vi "LVPortSetObjectMapNamepathDataToVartiant.vi"(0 "Type (or value to update)":variant, 1 "MatlabDataBundle":T1, 2 "NamePath":string[](array[string]), 3 "Namepath Index":i32, 6 "Allow Variant Values (f)":bool, 18 "Info":string[](array[string])) -> (14 "Value":variant)   [LabVIEW 2017]
uses:
  LVPortObjectMapNamepathData.ctl
  LVPortObjectMapDataTypeEnum.ctl
  LVPortObjectMapContainerTypeEnum.ctl
panel:
  out "Updating index":i32
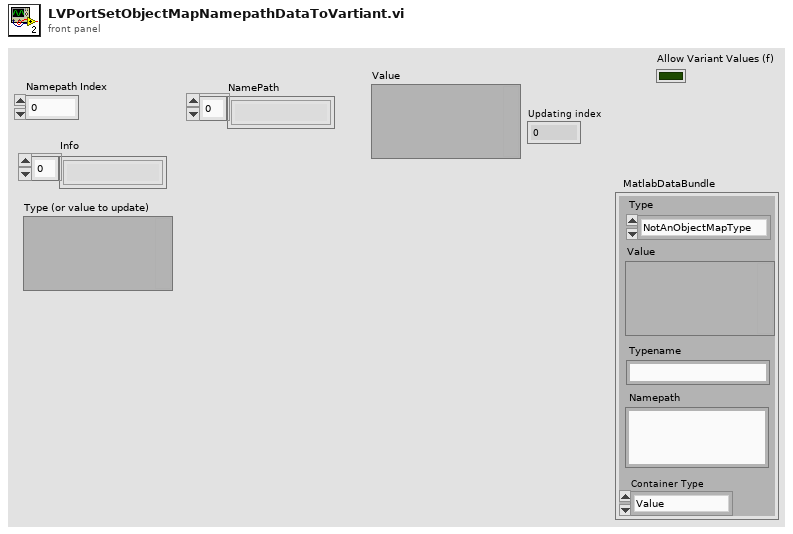
[diagram p1: front panel]
types:
  T1 = typedef "LVPortObjectMapNamepathData.ctl" = cluster{"Type":T2, "Value":variant, "Namepath":string, "Typename":string, "Container Type":T3}
  T2 = typedef "LVPortObjectMapDataTypeEnum.ctl" = enum16{"NotAnObjectMapType", "Real", "Complex", "String", "Boolean"}
  T3 = typedef "LVPortObjectMapContainerTypeEnum.ctl" = enum16{"Value", "Array", "Waveform"}
  T4 = typedef "NI_Data Type.lvlib/Data Type.ctl" = enum8{"Invalid Type", "Void", "I8", "I16", "I32", "I64", "U8", "U16", "U32", "U64", "Single Float", "Double Float", "Extended Float", "Single Complex", "Double Complex", "Extended Complex", "Enum U8", "Enum U16", "Enum U32", "Enum U64", "Single Float With Unit", "Double Float With Unit", "Extended Float With Unit", "Single Complex with Unit", "Double Complex with Unit", "Extended Complex with Unit", "Boolean", "String", "Path", "Picture", "Tag", "Array", "Cluster", "Variant", "LV Variant", "Waveform", "Timestamp", "Digital Waveform", "Digital Data", "ExpressData", "Refnum", "External Data", "VI", "Poly VI", "LabVIEW Class Instance", "Fixed Point"}
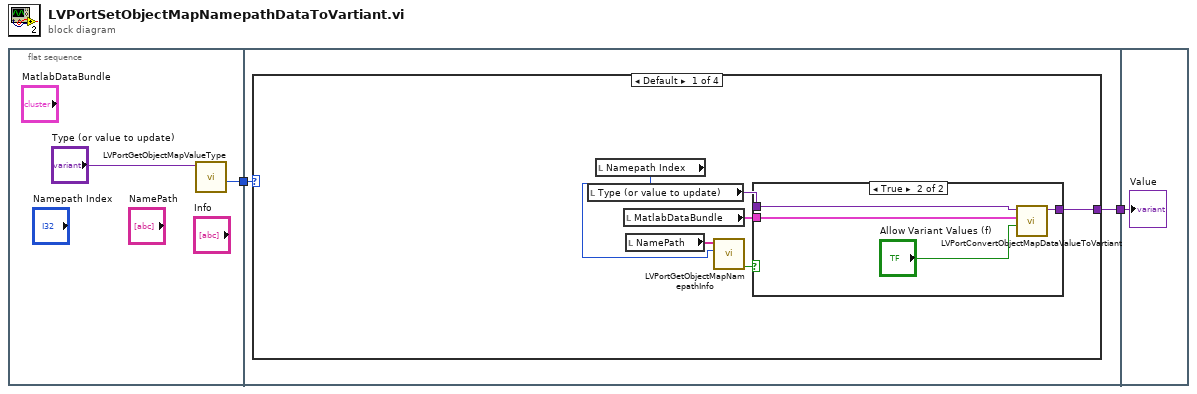
[diagram p0: block diagram]
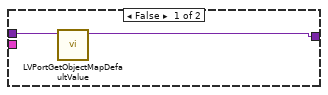
[diagram p2: hidden frame]
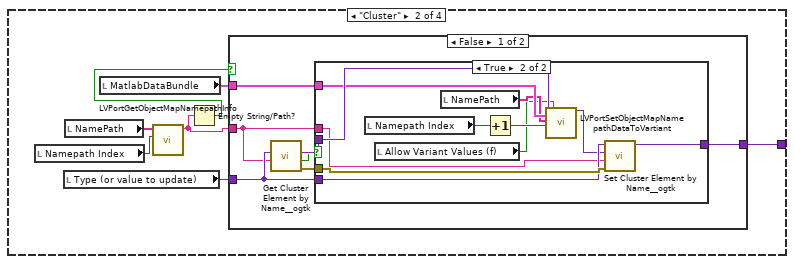
[diagram p3: hidden frame]
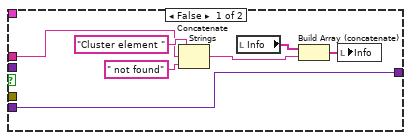
[diagram p4: hidden frame]
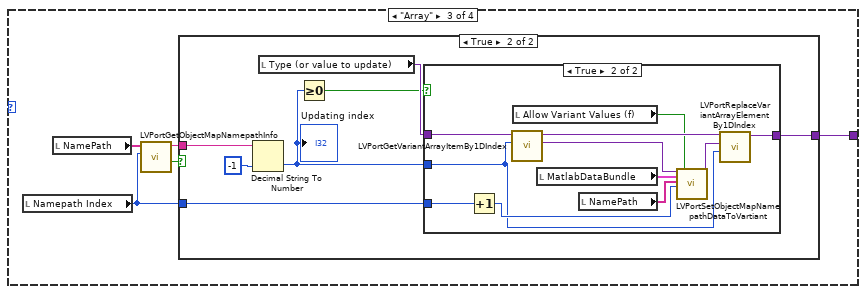
[diagram p6: hidden frame]
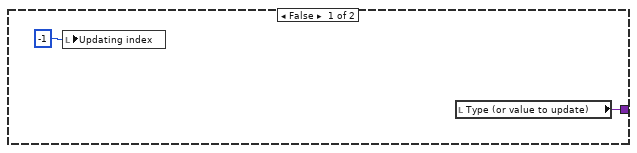
[diagram p7: hidden frame]
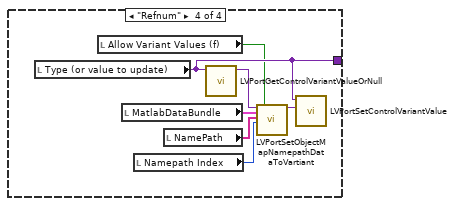
[diagram p9: hidden frame]
diagram:
  n1 = flat-sequence {
    tunnel: [w3] -> w2
    tunnel: w2 -> [w5]
    tunnel: [w6] -> w1
    tunnel: w1 -> [w85]
    frame #0 {
      n2 = call "LVPortGetObjectMapValueType.vi"("Value"="Type (or value to update)") -> ("Type"=w3:T4)  [unwired: 6 in, 4 out]
    }
    frame #1 {
      n3 = case shown="Default" w5 {
        tunnel: [w12 w23 w56 w82] -> w6
        frame Default {
          n4 = local read "Type (or value to update)"() -> (w11:variant)
          n5 = local read "Namepath Index"() -> (w9:i32)
          n6 = local read "MatlabDataBundle"() -> (w10:T1)
          n7 = local read "NamePath"() -> (w8:string[])
          n8 = call "LVPortGetObjectMapNamepathInfo.vi"("Namepath Index"=w9, "NamePath"=w8) -> ("At path end"=w7:bool)  [unwired: 7 in, 2 out]
          n9 = case shown="True" w7 {
            tunnel: [w14 w18] -> w12
            tunnel: w11 -> [w13 w17]
            tunnel: w10 -> [_ w16]
            frame False {
              n10 = call "LVPortGetObjectMapDefaultValue.vi"("From Value Type"=w13) -> ("Default Value"=w14:variant)  [unwired: 10 in]
            }
            frame True {
              n11 = call "LVPortConvertObjectMapDataValueToVartiant.vi"("Allow Variant Values (f)"="Allow Variant Values (f)", "MatlabDataBundle"=w16, "Data Value"=w17) -> ("Value"=w18:variant)  [unwired: 8 in]
            }
          }
        }
        frame "Cluster" {
          n12 = local read "Namepath Index"() -> (w19:i32)
          n13 = local read "Type (or value to update)"() -> (w24:variant)
          n14 = local read "NamePath"() -> (w21:string[])
          n15 = local read "MatlabDataBundle"() -> (w25:T1)
          n16 = call "LVPortGetObjectMapNamepathInfo.vi"("Namepath Index"=w19, "NamePath"=w21) -> ("Name"=w20:string)  [unwired: 7 in, 2 out]
          n17 = Empty String/Path?(string/path=w20) -> (empty?=w22:bool)
          n18 = case shown="False" w22 {
            tunnel: w25 -> [w31 _]
            tunnel: w24 -> [w29 w51]
            tunnel: [w28 w51] -> w23
            tunnel: w20 -> [w27 _]
            frame False {
              n19 = call <userlib>:"Get Cluster Element by Name__ogtk.vi"("Element Name"=w27, "Cluster"=w29) -> ("error out"=w30:errorcluster, "found?"=w26:bool, "VElement"=w32:variant)  [unwired: 7 in]
              n20 = case shown="True" w26 {
                tunnel: w32 -> [_ w50]
                tunnel: w31 -> [_ w49]
                tunnel: w30 -> [_ w48]
                tunnel: w29 -> [w39 w47]
                tunnel: [w39 w46] -> w28
                tunnel: w27 -> [w35 w44]
                frame False {
                  n21 = Concatenate Strings("Cluster element ", w35, " not found") -> (w37:string)
                  n22 = local read "Info"() -> (w38:string[])
                  n23 = Build Array (concatenate)(w38, w37) -> (w33:string[])
                  n24 = local write "Info"(w33) -> ()
                }
                frame True {
                  n25 = local read "Namepath Index"() -> (w42:i32)
                  n26 = local read "Allow Variant Values (f)"() -> (w40:bool)
                  n27 = local read "NamePath"() -> (w43:string[])
                  n28 = Increment(x=w42) -> (x+1=w41:i32)
                  n29 = call "LVPortSetObjectMapNamepathDataToVartiant.vi"("Type (or value to update)"=w50, "MatlabDataBundle"=w49, "NamePath"=w43, "Namepath Index"=w41, "Allow Variant Values (f)"=w40) -> ("Value"=w45:variant)  [unwired: 14 in]
                  n30 = call <userlib>:"Set Cluster Element by Name__ogtk.vi"("error in (no error)"=w48, "Element Name (\"\": New Element Data Name)"=w44, "New Element Value"=w45, "Cluster"=w47) -> ("VCluster out"=w46:variant)  [unwired: 5 in, 2 out]
                }
              }
            }
            frame True {
            }
          }
        }
        frame "Array" {
          n31 = local read "Namepath Index"() -> (w55:i32)
          n32 = local read "NamePath"() -> (w54:string[])
          n33 = call "LVPortGetObjectMapNamepathInfo.vi"("Namepath Index"=w55, "NamePath"=w54) -> ("Namepart found?"=w52:bool, "Name"=w53:string)  [unwired: 7 in, 1 out]
          n34 = case shown="True" w52 {
            tunnel: [w58 w64] -> w56
            tunnel: w55 -> [_ w60]
            tunnel: w53 -> [_ w59]
            frame False {
              n35 = local write "Updating index"(-1 ("Updating index")) -> ()
              n36 = local read "Type (or value to update)"() -> (w58:variant)
            }
            frame True {
              n37 = Decimal String To Number(string=w59, default (0L)=-1 ("default (0 I32)")) -> (number=w62:i32)  [unwired: 1 in, 1 out]
              "Updating index" <- w62
              n38 = local read "Type (or value to update)"() -> (w65:variant)
              n39 = Greater Or Equal To 0?(x=w62) -> (x >= 0?=w61:bool)
              n40 = case shown="True" w61 {
                tunnel: w65 -> [w66 w77]
                tunnel: w62 -> [_ w68]
                tunnel: [w66 w71] -> w64
                tunnel: w60 -> [_ w70]
                frame False {
                }
                frame True {
                  n41 = Increment(x=w70) -> (x+1=w69:i32)
                  n42 = call "LVPortGetVariantArrayItemBy1DIndex.vi"("Index"=w68, "Array in"=w77) -> ("Array Element"=w74:variant, "Array out"=w72:variant)  [unwired: 8 in]
                  n43 = local read "Allow Variant Values (f)"() -> (w67:bool)
                  n44 = local read "MatlabDataBundle"() -> (w75:T1)
                  n45 = local read "NamePath"() -> (w76:string[])
                  n46 = call "LVPortSetObjectMapNamepathDataToVartiant.vi"("Type (or value to update)"=w74, "MatlabDataBundle"=w75, "NamePath"=w76, "Namepath Index"=w69, "Allow Variant Values (f)"=w67) -> ("Value"=w73:variant)  [unwired: 14 in]
                  n47 = call "LVPortReplaceVariantArrayElementBy1DIndex.vi"("Index (1D)"=w68, "Value"=w73, "Array in"=w72) -> ("Array out"=w71:variant)  [unwired: 8 in]
                }
              }
            }
          }
        }
        frame "Refnum" {
          n48 = local read "Type (or value to update)"() -> (w82:variant)
          n49 = local read "Allow Variant Values (f)"() -> (w78:bool)
          n50 = local read "MatlabDataBundle"() -> (w81:T1)
          n51 = local read "Namepath Index"() -> (w79:i32)
          n52 = local read "NamePath"() -> (w80:string[])
          n53 = call "LVPortGetControlVariantValueOrNull.vi"("ControlVariant"=w82) -> ("Value"=w84:variant)  [unwired: 9 in, 1 out]
          n54 = call "LVPortSetObjectMapNamepathDataToVartiant.vi"("Type (or value to update)"=w84, "MatlabDataBundle"=w81, "NamePath"=w80, "Namepath Index"=w79, "Allow Variant Values (f)"=w78) -> ("Value"=w83:variant)  [unwired: 14 in]
          n55 = call "LVPortSetControlVariantValue.vi"("Value"=w83, "ControlVariant"=w82) -> ()  [unwired: 9 in, 1 out]
        }
      }
    }
    frame #2 {
      "Value" <- w85
    }
  }
